vi "GetParam.vi"(8 "error in (no error)":errorcluster caption="entrée d'erreur (pas d'erreur)", 11 "SimpleImputer.lvclass":refnum<class "SimpleImputer.lvclass">) -> (0 "error out":errorcluster caption="sortie d'erreur", 2 "SimpleImputer":T1={"missing_values"="nan", "strategy"="mean", "fill_value"={"dtype"="", "str"="None", "int"=0}, "verbose"=0, "copy"=TRUE, "add_indicator"=FALSE}, 3 "SimpleImputer.lvclass":refnum<class "SimpleImputer.lvclass">)   [LabVIEW 2020, in "SimpleImputer.lvclass"]
doc: "Get Parameters"
uses:
  SimpleImputer.lvclass
  SimpleImputer.lvclass/SimpleImputer.ctl
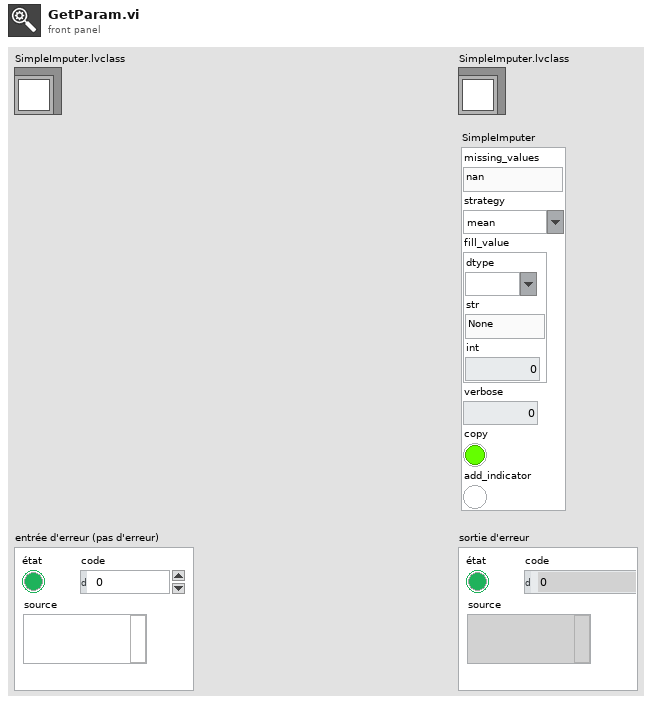
[diagram p1: front panel]
types:
  T1 = cluster{"missing_values":string, "strategy":string, "fill_value":cluster{"dtype":string, "str":string, "int":i32}, "verbose":i32, "copy":bool, "add_indicator":bool}
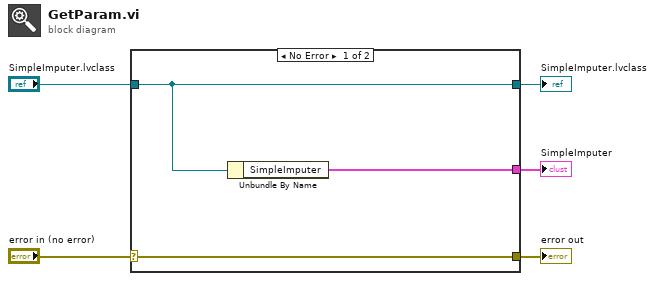
[diagram p0: block diagram]
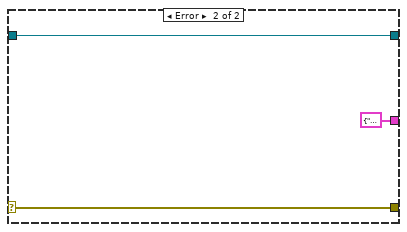
[diagram p2: hidden frame]
diagram:
  n1 = case shown="No Error" "error in (no error)" {
    selector: "error in (no error)" -> [w8 w10]
    tunnel: [w8 w10] -> w4
    tunnel: [w7 w11] -> w2
    tunnel: "SimpleImputer.lvclass" -> [w7 w11]
    tunnel: [w6 T1 {"missing_values"="", "strategy"="", "fill_value"={"dtype"="", "str"="", "int"=0}, "verbose"=0, "copy"=FALSE, "add_indicator"=FALSE} ("SimpleImputer")] -> w1
    frame No Error {
      n2 = Unbundle By Name(w7) -> ("SimpleImputer"=w6:T1)
    }
    frame Error {
    }
  }
  "error out" <- w4
  "SimpleImputer.lvclass" <- w2
  "SimpleImputer" <- w1
